vi "num216bit.vi"(11 "Trial#":u16) -> (3 "phd_array":bool[](array[boolean]))   [LabVIEW 2014]
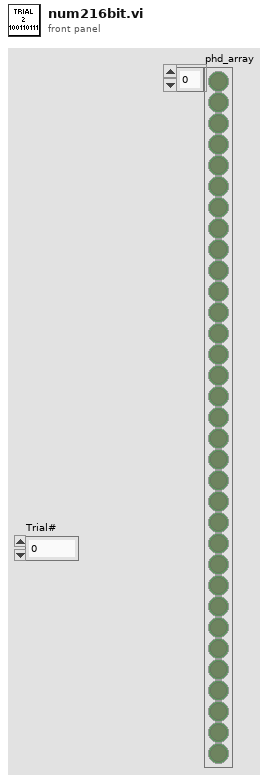
[diagram p1: front panel]
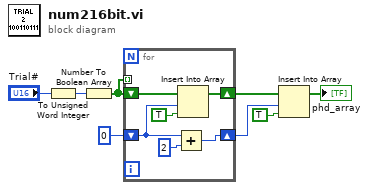
[diagram p0: block diagram]
diagram:
  n1 = To Unsigned Word Integer(number="Trial#") -> (unsigned 16bit integer=w1:u16)
  n2 = Number To Boolean Array(number=w1) -> (Boolean array=w7:bool[])
  n3 = for {
    tunnel: w7 -> [_] mode=indexing
    shift-right: [w13] -> w3
    shift-left: 0 -> [w9]
    shift-right: [w11] -> w5
    shift-left: w7 -> [w12]
    n4 = Add(x=w9, y=2) -> (x+y=w13:i32)
    n5 = Insert Into Array(array=w12, index=w9, new element=TRUE) -> (w11:bool[])
  }
  n6 = Insert Into Array(array=w5, index=w3, new element=TRUE) -> (→"phd_array":bool[])
